vi "ce14.BCC.vi"(8 "error in (no error)":errorcluster, 11 "mess in":string) -> (0 "error out":errorcluster, 1 "BCC":string, 3 "mess out":string)   [LabVIEW 2018, in "CE14_eMIC.lvlib"]
uses:
  CE14_eMIC.lvlib
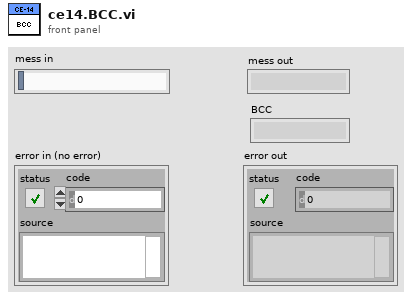
[diagram p1: front panel]
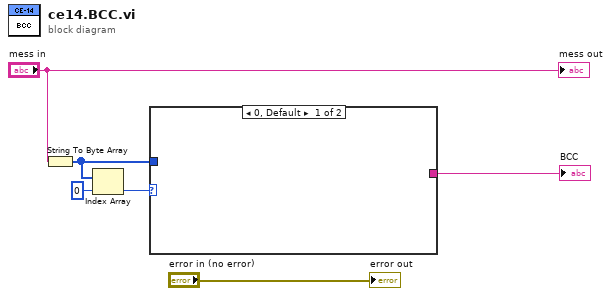
[diagram p0: block diagram]
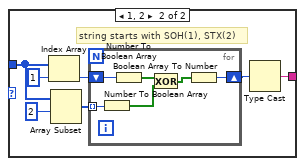
[diagram p2: hidden frame]
diagram:
  n1 = String To Byte Array(string="mess in") -> (unsigned byte array=w4:u8[])
  n2 = Index Array(array=w4, index=0) -> (element=w3:u8)
  n3 = case shown="0, Default" w3 {
    tunnel: [_ w9] -> w5
    tunnel: w4 -> [_ w7]
    frame 0, Default {
    }
    frame 1, 2 {
      # "string starts with SOH(1), STX(2)"
      n4 = Index Array(array=w7, index=1) -> (element=w13:u8)
      n5 = Array Subset(array=w7, index=2) -> (w11:u8[])  [unwired: 1 in]
      n6 = for {
        shift-right: [w14] -> w8
        shift-left: w13 -> [w19]
        tunnel: w11 -> [w18] mode=indexing
        n7 = Number To Boolean Array(number=w18) -> (Boolean array=w17:bool[])
        n8 = Number To Boolean Array(number=w19) -> (Boolean array=w16:bool[])
        n9 = Exclusive Or(1:w17, 2:w16) -> (0:w15:bool[])
        n10 = Boolean Array To Number(Boolean array=w15) -> (number=w14:u8)
      }
      n11 = Type Cast(x=w8) -> (*(type *) &x=w9:string)  [unwired: 1 in]
    }
  }
  "BCC" <- w5
  "error out" <- "error in (no error)"
  "mess out" <- "mess in"
